vi "Week2_Slide14_ResetCounter.vi"() -> ()   [LabVIEW 2015]
panel:
  in  "Reset":bool
  out "Counter":dbl
  in  "stop":bool
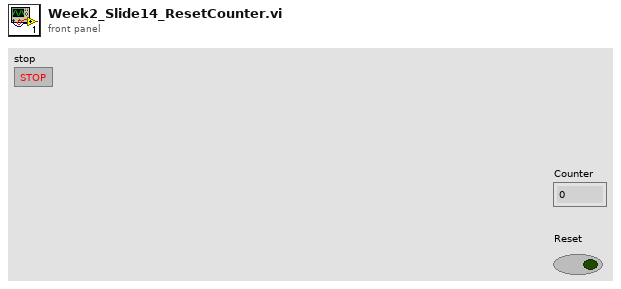
[diagram p1: front panel]
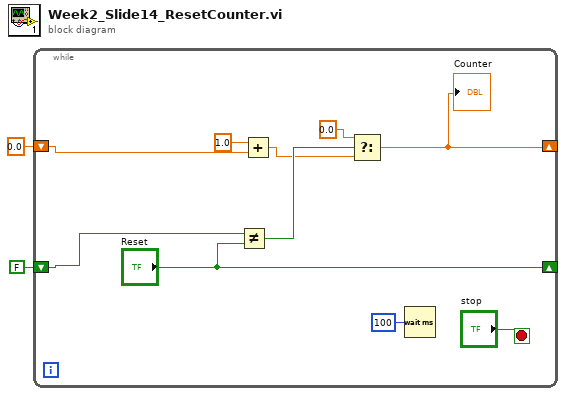
[diagram p0: block diagram]
diagram:
  n1 = while {
    shift-right: [w5] -> _
    shift-left: 0.0 -> [w10]
    shift-right: ["Reset"] -> _
    shift-left: FALSE ("Reset") -> [w7]
    stop <- "stop" stop-if-true
    n2 = Not Equal?(x=w7, y="Reset") -> (x != y?=w6:bool)
    n3 = Add(x=1.0, y=w10) -> (x+y=w4:dbl)
    n4 = Select(t=0.0 ("f"), s=w6, f=w4) -> (s? t:f=w5:dbl)
    "Counter" <- w5
    n5 = Wait (ms)(milliseconds to wait=u32 100) -> ()  [unwired: 1 out]
  }
